vi "Read Map - Enemy Position.vi"(8 "distance (10)":i32=10, 9 "column":i32, 10 "row":i32, 11 "map in":refnum<data-value>) -> (0 "found?":bool, 1 "enemy column":i32, 2 "enemy row":i32, 3 "map out":refnum<data-value>, 4 "number of enemies":i32)   [LabVIEW 2015, in "DS Square.lvlib"]
uses:
  DS Square.lvlib
  Square/Square.lvclass
  Square State.ctl
  Square Status.ctl
  Map.ctl
  Center of Mass.ctl
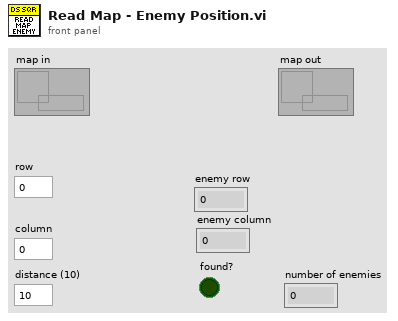
[diagram p1: front panel]
types:
  T1 = typedef "DS Square.lvlib/Square State.ctl" = enum16{"Unknown", "Empty", "Occupied - Active", "Occupied - Cool Down", "Attacked", "Enemy", "Enemy Wall"}
  T2 = typedef "DS Square.lvlib/Map.ctl" = cluster{"squares":T3[][], "center of mass":T4}
  T3 = typedef "DS Square.lvlib/Square Status.ctl" = cluster{"square state":T1, "probability":dbl, "last update":i32}
  T4 = typedef "DS Square.lvlib/Center of Mass.ctl" = cluster{"row":dbl, "col":dbl, "mass":dbl}
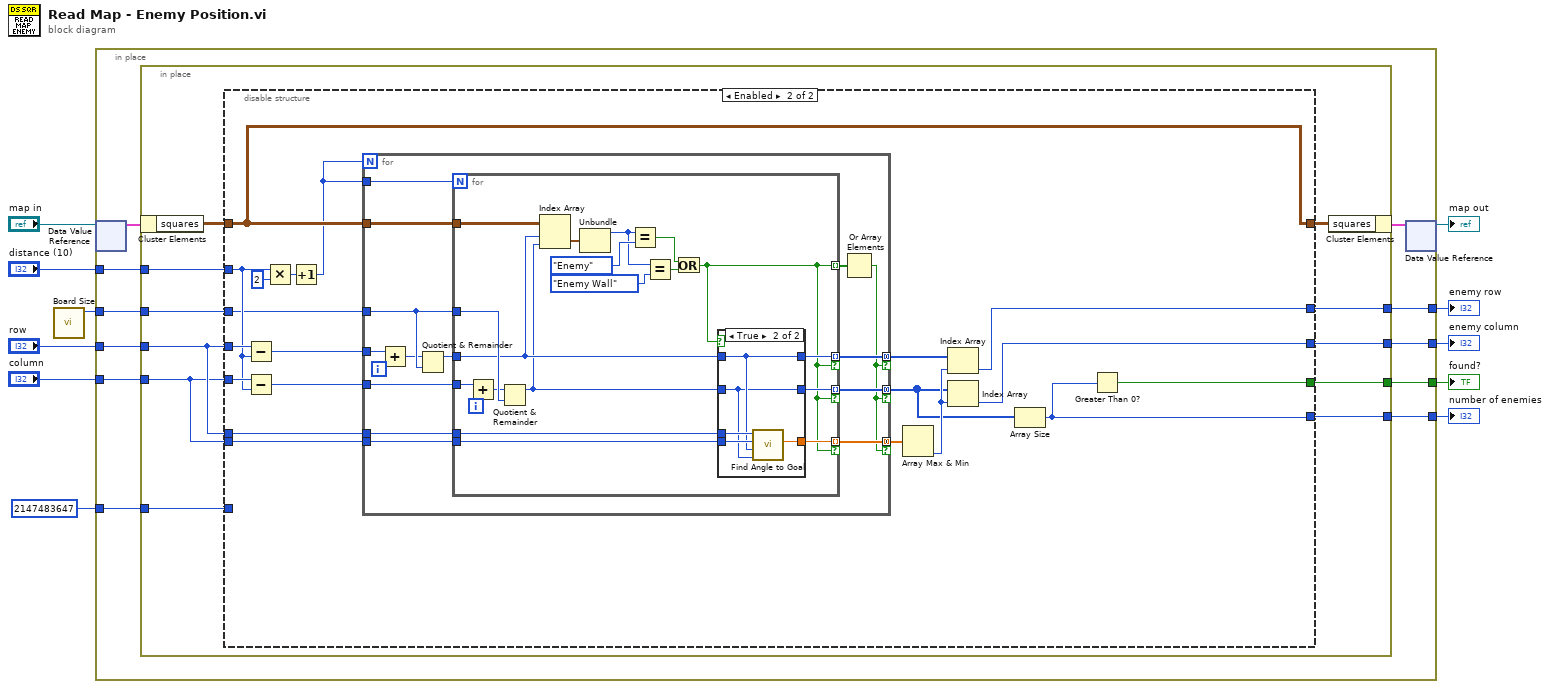
[diagram p0: block diagram]
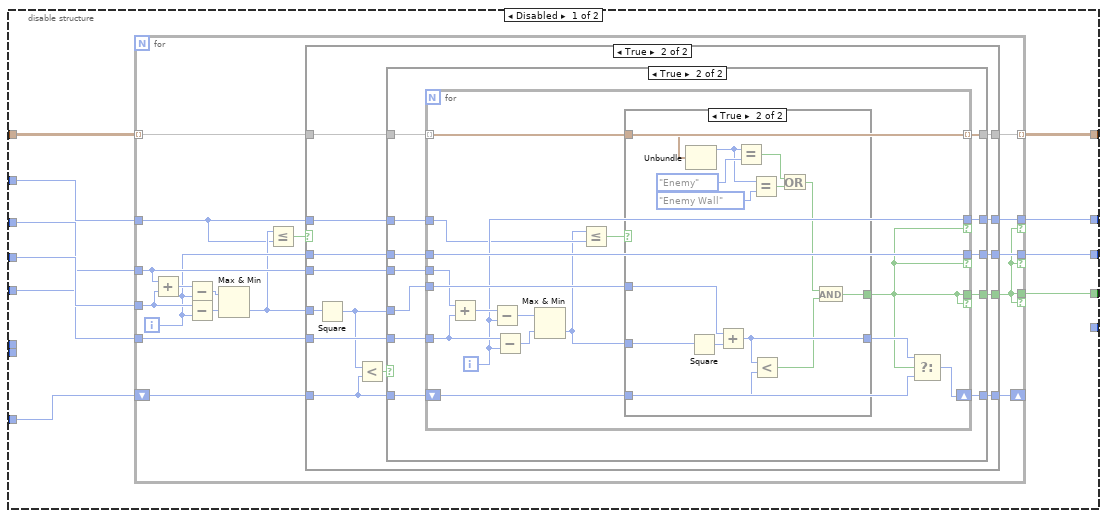
[diagram p2: hidden frame]
diagram:
  n1 = call "Board Size.vi"() -> ("Board Size"=w6:i32)  [unwired: 11 in]
  n2 = in-place {
    in-place-border: "row" -> [w20]
    in-place-border: 2147483647 ("column") -> [w19]
    in-place-border: "column" -> [w18]
    in-place-border: w6 -> [w17]
    in-place-border: [w16] -> w5
    in-place-border: [w15] -> w4
    in-place-border: [w14] -> w3
    in-place-border: "distance (10)" -> [w13]
    in-place-border: [w12] -> w1
    n3 = in-place-dvr #1("map in") -> (w22:T2)  [unwired: 1 out]
    n4 = in-place {
      in-place-border: w20 -> [w25]
      in-place-border: w19 -> [w31]
      in-place-border: w18 -> [w24]
      in-place-border: w17 -> [w30]
      in-place-border: [w29] -> w16
      in-place-border: [w28] -> w15
      in-place-border: [w27] -> w14
      in-place-border: w13 -> [w26]
      in-place-border: [w23] -> w12
      n5 = in-place-cluster #2(w22) -> ("squares"=w33:T3[][])
      n6 = disable-structure shown="Enabled" {
        disable-tunnel: w33 -> [w43 w139]
        disable-tunnel: [w42 w139] -> w32
        disable-tunnel: w25 -> [w41 w137]
        disable-tunnel: w31 -> [w40 _]
        disable-tunnel: w24 -> [w39 w136]
        disable-tunnel: w30 -> [w38 w133]
        disable-tunnel: [w37 w126] -> w29
        disable-tunnel: [w36 w125] -> w28
        disable-tunnel: [w35 w123] -> w27
        disable-tunnel: w26 -> [w34 w135]
        disable-tunnel: w25 -> [_ w131]
        disable-tunnel: w24 -> [_ w130]
        disable-tunnel: [_ w122] -> w23
        frame Disabled {
          n7 = for {
            tunnel: w43 -> [w60] mode=indexing
            tunnel: [w59] -> w42 mode=indexing
            tunnel: w41 -> [w55]
            shift-right: [w58] -> _
            shift-left: w40 -> [w56]
            tunnel: w39 -> [w57]
            tunnel: w38 -> [w51]
            tunnel: [w49] -> w36 if=w47
            tunnel: [w48] -> w37 if=w47
            tunnel: [w47] -> w35 if=w47
            tunnel: w34 -> [w44]
            i -> [w50]
            n8 = Add(x=w51, y=w55) -> (x+y=w54:i32)
            n9 = Subtract(x=w54, y=w50) -> (x-y=w53:i32)
            n10 = Subtract(x=w55, y=w50) -> (x-y=w52:i32)
            n11 = Max & Min(x=w53, y=w52) -> (min(x,y)=w46:i32)  [unwired: 1 out]
            n12 = Less Or Equal?(x=w46, y=w44) -> (x <= y?=w45:bool)
            n13 = case shown="True" w45 {
              tunnel: w60 -> [w62 w76]
              tunnel: [w62 w75] -> w59
              tunnel: [w61 w74] -> w58
              tunnel: w57 -> [_ w73]
              tunnel: w56 -> [w61 w71]
              tunnel: w46 -> [_ w69]
              tunnel: w51 -> [_ w68]
              tunnel: w50 -> [_ w67]
              tunnel: [_ w66] -> w49
              tunnel: [_ w65] -> w48
              tunnel: [_ w64] -> w47
              tunnel: w44 -> [_ w63]
              frame False {
              }
              frame True {
                n14 = Square(x=w69) -> (x^2=w72:i32)
                n15 = Less?(x=w72, y=w71) -> (x < y?=w70:bool)
                n16 = case shown="True" w70 {
                  tunnel: w76 -> [w79 w91]
                  tunnel: [w79 w90] -> w75
                  tunnel: [w78 w89] -> w74
                  tunnel: w73 -> [_ w88]
                  tunnel: w72 -> [_ w87]
                  tunnel: w71 -> [w78 w86]
                  tunnel: w68 -> [_ w85]
                  tunnel: w67 -> [w77 w84]
                  tunnel: [w77 w83] -> w66
                  tunnel: [_ w82] -> w64
                  tunnel: [_ w81] -> w65
                  tunnel: w63 -> [_ w80]
                  frame False {
                  }
                  frame True {
                    n17 = for {
                      tunnel: w91 -> [w107] mode=indexing
                      tunnel: [w107] -> w90 mode=indexing
                      shift-right: [w103] -> w89
                      shift-left: w86 -> [w105]
                      tunnel: w88 -> [w101]
                      tunnel: w87 -> [w106]
                      tunnel: w85 -> [w102]
                      tunnel: w84 -> [w97]
                      tunnel: [w97] -> w83 if=w95
                      tunnel: [w95] -> w82 if=w95
                      tunnel: [w96] -> w81 if=w95
                      tunnel: w80 -> [w94]
                      i -> [w96]
                      n18 = Add(x=w102, y=w101) -> (x+y=w100:i32)
                      n19 = Subtract(x=w100, y=w96) -> (x-y=w99:i32)
                      n20 = Subtract(x=w101, y=w96) -> (x-y=w98:i32)
                      n21 = Max & Min(x=w99, y=w98) -> (min(x,y)=w93:i32)  [unwired: 1 out]
                      n22 = Less Or Equal?(x=w93, y=w94) -> (x <= y?=w92:bool)
                      n23 = case shown="True" w92 {
                        tunnel: w107 -> [_ w120]
                        tunnel: w106 -> [_ w114]
                        tunnel: w105 -> [_ w113]
                        tunnel: [_ w112] -> w104
                        tunnel: w93 -> [_ w111]
                        tunnel: [_ w108] -> w95
                        frame False {
                        }
                        frame True {
                          n24 = Unbundle(w120) -> ("square state"=w118:T1)  [unwired: 2 out]
                          n25 = Square(x=w111) -> (x^2=w115:i32)
                          n26 = Add(x=w114, y=w115) -> (x+y=w112:i32)
                          n27 = Equal?(x=w118, y=Square_State."Enemy" ("square state")) -> (x = y?=w117:bool)
                          n28 = Equal?(x=w118, y=Square_State."Enemy Wall" ("square state")) -> (x = y?=w116:bool)
                          n29 = Less?(x=w112, y=w113) -> (x < y?=w109:bool)
                          n30 = Or(x=w117, y=w116) -> (x .or. y?=w110:bool)
                          n31 = And(x=w110, y=w109) -> (x .and. y?=w108:bool)
                        }
                      }
                      n32 = Select(t=w104, s=w95, f=w105) -> (s? t:f=w103:i32)
                    }
                  }
                }
              }
            }
          }
        }
        frame Enabled {
          n33 = Subtract(x=w137, y=w135) -> (x-y=w134:i32)
          n34 = Subtract(x=w136, y=w135) -> (x-y=w132:i32)
          n35 = Multiply(x=w135, y=2) -> (x*y=w140:i32)
          n36 = Increment(x=w140) -> (x+1=w138:i32)
          n37 = for {
            N: w138 -> [_]
            tunnel: w139 -> [w155]
            tunnel: w138 -> [w156]
            tunnel: w134 -> [w151]
            tunnel: w133 -> [w153]
            tunnel: w132 -> [w152]
            tunnel: w131 -> [w148]
            tunnel: w130 -> [w147]
            tunnel: [w146] -> w128 mode=concatenating if=w142
            tunnel: [w145] -> w124 mode=concatenating if=w142
            tunnel: [w144] -> w129 mode=concatenating if=w142
            i -> [w149]
            n38 = Add(x=w151, y=w149) -> (x+y=w150:i32)
            n39 = Quotient & Remainder(x=w150, y=w153) -> (x-y*floor(x/y)=w154:i32)  [unwired: 1 out]
            n40 = for {
              N: w156 -> [_]
              tunnel: w155 -> [w174]
              tunnel: w154 -> [w162]
              tunnel: w153 -> [w175]
              tunnel: w152 -> [w167]
              tunnel: w148 -> [w164]
              tunnel: w147 -> [w163]
              tunnel: [w160] -> w144 mode=indexing if=w157
              tunnel: [w159] -> w146 mode=indexing if=w157
              tunnel: [w158] -> w145 mode=indexing if=w157
              tunnel: [w157] -> w143 mode=indexing
              i -> [w165]
              n41 = Add(x=w167, y=w165) -> (x+y=w166:i32)
              n42 = Quotient & Remainder(x=w166, y=w175) -> (x-y*floor(x/y)=w161:i32)  [unwired: 1 out]
              n43 = Index Array(array=w174, index (row)=w162, index (col)=w161) -> (element=w168:T3)
              n44 = Unbundle(w168) -> ("square state"=w171:T1)  [unwired: 2 out]
              n45 = Equal?(x=w171, y=Square_State."Enemy" ("square state")) -> (x = y?=w170:bool)
              n46 = Equal?(x=w171, y=Square_State."Enemy Wall" ("square state")) -> (x = y?=w169:bool)
              n47 = Or(x=w170, y=w169) -> (x .or. y?=w157:bool)
              n48 = case shown="True" w157 {
                tunnel: w164 -> [_ w180]
                tunnel: w163 -> [_ w179]
                tunnel: w162 -> [_ w177]
                tunnel: w161 -> [_ w176]
                tunnel: [_ w178] -> w160
                tunnel: [_ w177] -> w159
                tunnel: [_ w176] -> w158
                frame False {
                }
                frame True {
                  n49 = call "Find Angle to Goal.vi"("Goal Column"=w176, "Goal Row"=w177, "Column"=w179, "Row"=w180) -> ("distance"=w178:dbl)  [unwired: 4 in, 3 out]
                }
              }
            }
            n50 = Or Array Elements(Boolean array=w143) -> (logical OR=w142:bool)
          }
          n51 = Array Max & Min(array=w129) -> (min index (indices)=w127:i32)  [unwired: 3 out]
          n52 = Index Array(array=w128, index=w127) -> (element=w126:i32)
          n53 = Index Array(array=w124, index=w127) -> (element=w125:i32)
          n54 = Array Size(array=w124) -> (size(s)=w122:i32)
          n55 = Greater Than 0?(x=w122) -> (x > 0?=w123:bool)
        }
      }
      n56 = in-place-cluster #2("squares"=w32) -> (w21:T2)
    }
    n57 = in-place-dvr #1(w21) -> (→"map out":refnum<data-value>)  [unwired: 1 out]
  }
  "enemy row" <- w5
  "enemy column" <- w4
  "found?" <- w3
  "number of enemies" <- w1
